vi "updateGitRevision.vi"() -> ()   [LabVIEW 2017]
uses:
  <vilib>/Utility/traverseref.llb/TRef TravTarget.ctl
  <vilib>/Utility/traverseref.llb/VI Scripting - Traverse.lvlib
panel:
  out "path":path
  out "standard output":string
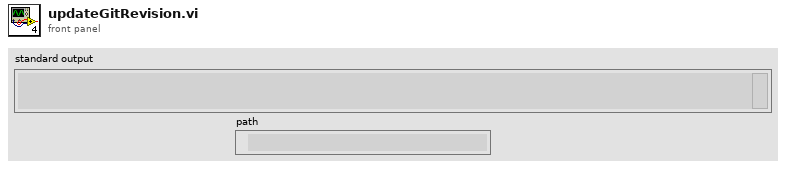
[diagram p1: front panel]
types:
  T1 = typedef "TRef TravTarget.ctl" = enum16{"FP", "BD", "Other"}
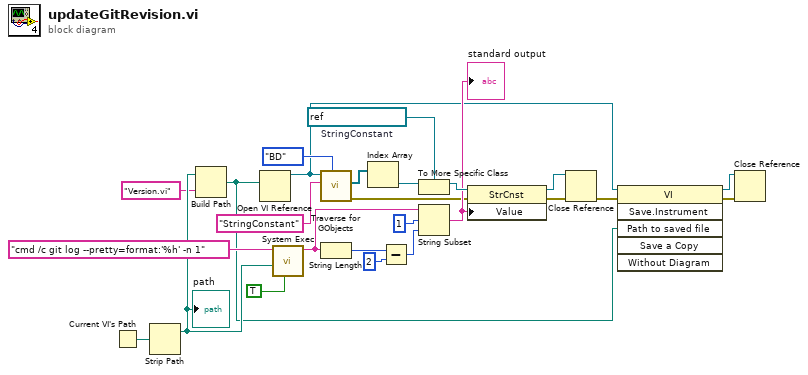
[diagram p0: block diagram]
diagram:
  w11 = refnum<vi> refnum  # StringConstant
  n1 = Current VI's Path() -> (path=w24:path)
  n2 = Strip Path(path=w24) -> (stripped path=w17:path)  [unwired: 1 out]
  "path" <- w17
  n3 = Build Path(base path=w17, name or relative path="Version.vi") -> (appended path=w3:path)
  n4 = Open VI Reference(vi path=w3) -> (vi reference=w4:refnum<vi>)  [unwired: 5 in, 1 out]
  n5 = call <vilib>:"System Exec.vi"("run minimized? (F)"=TRUE, "working directory"=w17, "command line"="cmd /c git log --pretty=format:'%h' -n 1") -> ("standard output"=w19:string)  [unwired: 5 in, 3 out]
  n6 = call <vilib>:"Traverse for GObjects.vi"("Traverse Target"=TRef_TravTarget."BD", "Class Name"="StringConstant", "VI Refnum"=w4) -> ("error out"=w8:errorcluster, "References"=w13:refnum<vi>[])  [unwired: 5 in, 2 out]
  n7 = String Length(string=w19) -> (length=w23:i32)
  n8 = Index Array(array=w13) -> (element=w12:refnum<vi>)  [unwired: 1 in]
  n9 = Subtract(x=w23, y=2) -> (x-y=w21:i32)
  n10 = To More Specific Class(target class=w11, reference=w12) -> (specific class reference=w10:refnum<vi>)  [unwired: 1 in, 1 out]
  n11 = String Subset(string=w19, offset (0)=1, length (rest)=w21) -> (substring=w9:string)
  "standard output" <- w9
  n12 = property class="StrCnst"(reference=w10, error in=w8, "Value"=w9) -> (reference out=w7:refnum<vi>, error out=w6:errorcluster)
  n13 = Close Reference(reference=w7, error in (no error)=w6) -> (error out=w5:errorcluster)
  n14 = invoke class="VI" method="Save.Instrument"(reference=w4, error in=w5, "Path to saved file"=w3) -> (reference out=w1:refnum<vi>, error out=w2:errorcluster)  [unwired: 3 in, 4 out]
  n15 = Close Reference(reference=w1, error in (no error)=w2) -> ()  [unwired: 1 out]
